vi "微积分作业.vi"() -> ()   [LabVIEW 2014]
uses:
  <vilib>/Analysis/2dsp.llb/Integral Method.ctl
  <vilib>/Analysis/8numeric.llb/1D Numeric Integration.vi
  <vilib>/Analysis/NI_AALPro.lvlib
panel:
  in  "Final Condition 2":dbl[](array[numeric])=[0.0] caption="最终条件" format="%#_6f"
  in  "Initial Condition 2":dbl[](array[numeric])=[0.0] caption="初始条件" format="%#_6f"
  in  "Final Condition":dbl[](array[numeric])=[0.0] caption="最终条件"
  in  "Initial Condition":dbl[](array[numeric])=[0.0] caption="初始条件"
  in  "integration method":T1 caption="积分方法" items=["梯形法则", "Simpson法则", "Simpson 3/8法则", "Bode法则"]
  out "XY图 3":cluster{dbl[], "dX/dt":dbl[]}(graph)
  out "XY图 2":cluster{dbl[], "Integral X":dbl[]}(graph)
  out "XY图":cluster{dbl[], dbl[]}(graph)
  out "dt":dbl=1.0 step=0.001 format="%0.4f"
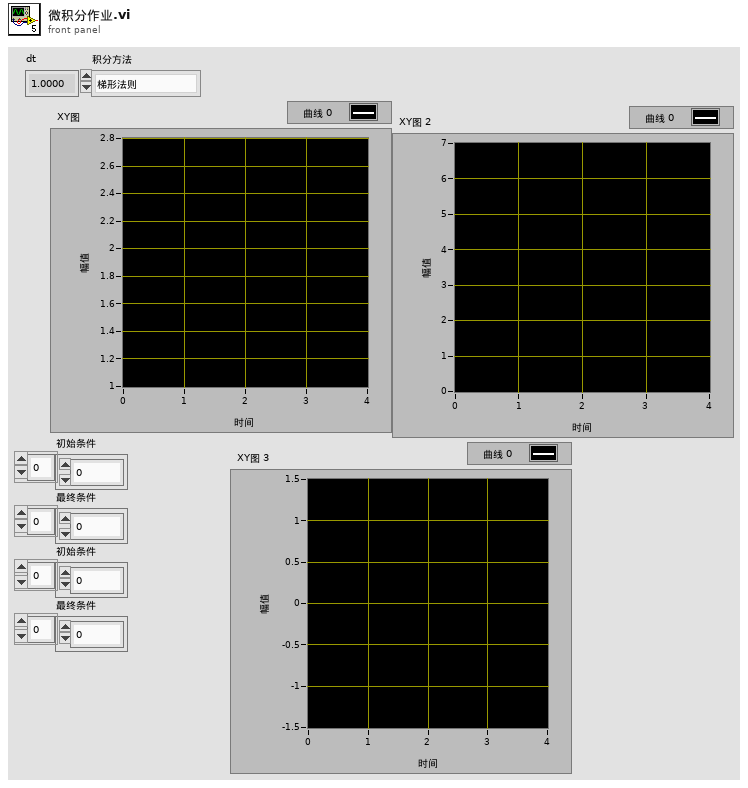
[diagram p1: front panel]
types:
  T1 = typedef "NI_AALPro.lvlib/Integral Method.ctl" = i32
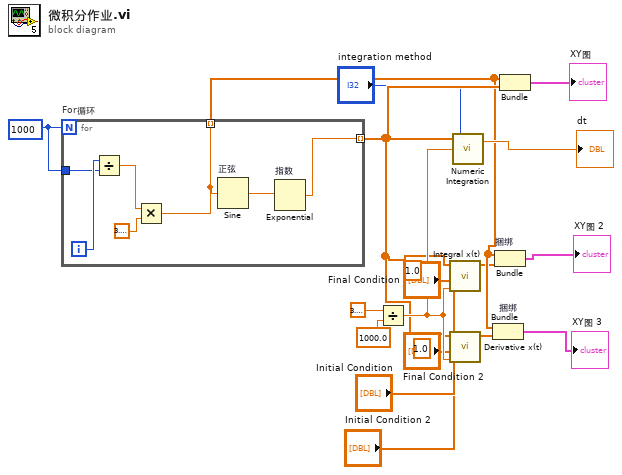
[diagram p0: block diagram]
diagram:
  (unwired) 1.0
  (unwired) 1.0
  w17 = 1000
  n1 = for "For循环" {
    N: w17 -> [_]
    tunnel: w17 -> [w23]
    tunnel: [w19] -> w11 mode=indexing
    tunnel: [w18] -> w10 mode=indexing
    i -> [w24]
    n2 = Divide(x=w24, y=w23) -> (x/y=w21:dbl)
    n3 = Multiply(x=w21, y=3.141592653589793) -> (x*y=w18:dbl)
    n4 = Sine "正弦"(x=w18) -> (sin(x)=w20:dbl)
    n5 = Exponential "指数"(1:w20) -> (0:w19:dbl)
  }
  n6 = Divide(x=3.141592653589793, y=1000.0) -> (x/y=w13:dbl)
  n7 = call <vilib>:"Integral x(t).vi"("dt"=w13, "Final Condition"="Final Condition", "Initial Condition"="Initial Condition", "X"=w11) -> ("Integral X"=w8:dbl[])  [unwired: 6 in, 1 out]
  n8 = call <vilib>:"Derivative x(t).vi"("dt"=w13, "Final Condition"="Final Condition 2", "Initial Condition"="Initial Condition 2", "X"=w11) -> ("dX/dt"=w9:dbl[])  [unwired: 6 in, 1 out]
  n9 = call-poly <vilib>:"Numeric Integration.vi"("integration method"="integration method", "dt"=w13, "Input Array"=w11) -> ("result"=→"dt":dbl)  [unwired: 1 out]
  n10 = Bundle "捆绑"(w10, "dX/dt"=w9) -> (→"XY图 3":cluster{dbl[], "dX/dt":dbl[]})  [unwired: 1 in]
  n11 = Bundle "捆绑"(w10, "Integral X"=w8) -> (→"XY图 2":cluster{dbl[], "Integral X":dbl[]})  [unwired: 1 in]
  n12 = Bundle(w10, w11) -> (→"XY图":cluster{dbl[], dbl[]})  [unwired: 1 in]
